vi "Write Com Port.vi"(8 "error in (no error)":errorcluster, 10 "Com Port":refnum<visa-resource-name>, 11 "SpinCoater in":refnum<class "SpinCoater.lvclass">) -> (0 "error out":errorcluster, 3 "SpinCoater out":refnum<class "SpinCoater.lvclass">)   [LabVIEW 2020, in "SpinCoater.lvclass"]
uses:
  <instrlib>/Classes/SpinCoater/SpinCoater.lvclass
  <instrlib>/Classes/SpinCoater/SpinCoater.lvclass/SpinCoater.ctl
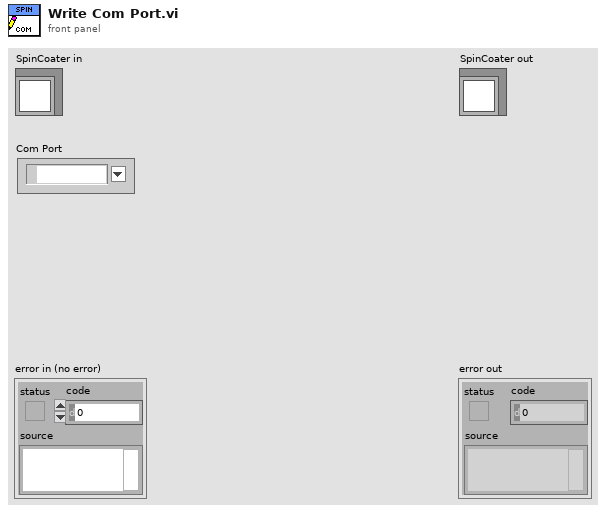
[diagram p1: front panel]
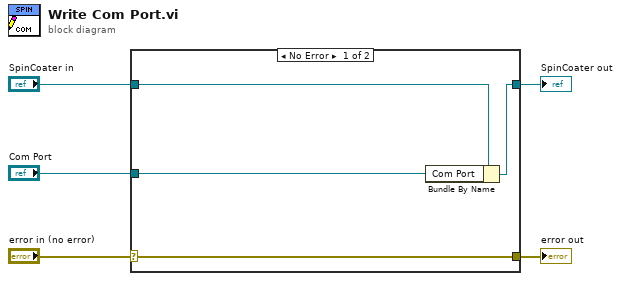
[diagram p0: block diagram]
diagram:
  n1 = case shown="No Error" "error in (no error)" {
    selector: "error in (no error)" -> [w9 w10]
    tunnel: [w9 w10] -> w4
    tunnel: [w7 w11] -> w2
    tunnel: "SpinCoater in" -> [w8 w11]
    tunnel: "Com Port" -> [w6 _]
    frame No Error {
      n2 = Bundle By Name(cluster=w8, "Com Port"=w6) -> (w7:refnum<class "SpinCoater.lvclass">)
    }
    frame Error {
    }
  }
  "error out" <- w4
  "SpinCoater out" <- w2
